vi "XY Graph Get Plot Properties.vi"(8 "Error In":errorcluster, 10 "Plot Idx":i32, 11 "XYGraph in":T1) -> (0 "Error Out":errorcluster, 2 "XY Plot Properties":T2, 3 "XYGraph out":T1, 4 "Plot.XScaleIdx":u32, 6 "Plot.YScaleIdx":u32)   [LabVIEW 2021, in "XY Graph Add-Ons.lvlib"]
uses:
  XY Graph Add-Ons.lvlib
  XY Graph Plot Properties.ctl
  XY Graph Refnum.ctl
panel:
  # "see the License on the block diagram (Ctrl+E or Window:Show Block Diagram)"
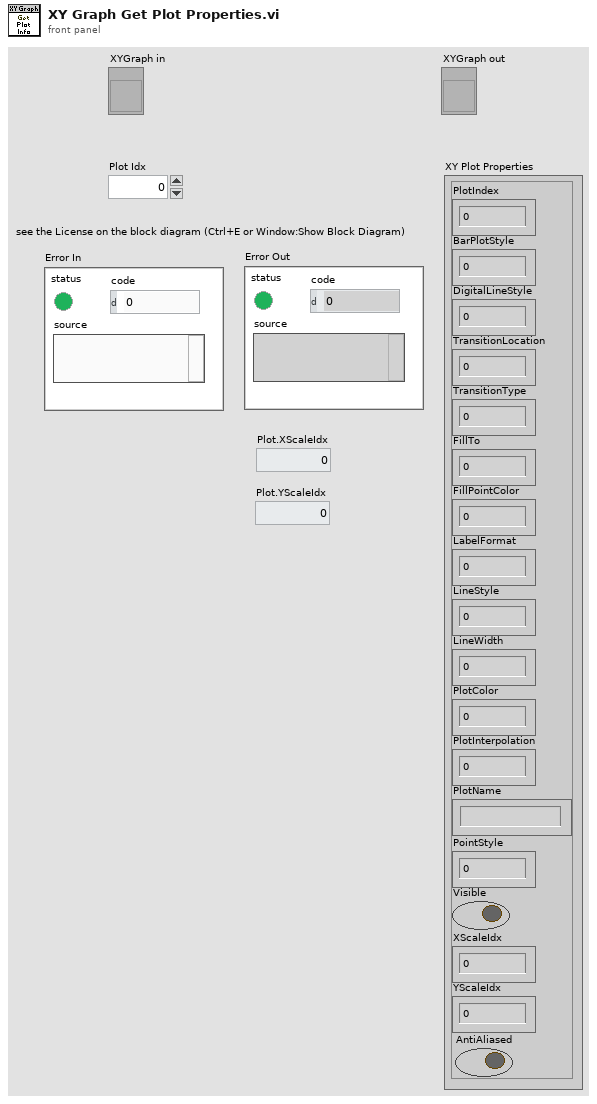
[diagram p1: front panel]
types:
  T1 = typedef "XY Graph Add-Ons.lvlib/XY Graph Refnum.ctl" = refnum<vi>
  T2 = typedef "XY Graph Add-Ons.lvlib/XY Graph Plot Properties.ctl" = cluster{"PlotIndex":i32, "BarPlotStyle":u8, "DigitalLineStyle":u8, "TransitionLocation":u8, "TransitionType":u8, "FillTo":i16, "FillPointColor":u32, "LabelFormat":u8, "LineStyle":u8, "LineWidth":u8, "PlotColor":u32, "PlotInterpolation":u8, "PlotName":string, "PointStyle":u8, "Visible":bool, "XScaleIdx":u32, "YScaleIdx":u32, "AntiAliased":bool}
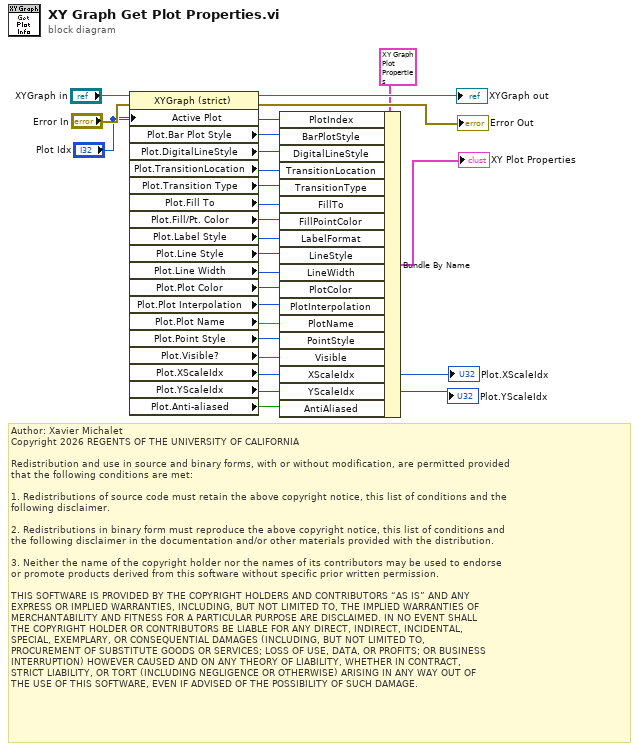
[diagram p0: block diagram]
diagram:
  # "Author: Xavier Michalet\nCopyright 2026 REGENTS OF THE UNIVERSITY OF CALIFORNIA\n\nRedistribution and use in source and binary forms, with or without modification, are permitted provided\nthat the following conditions are met:\n\n1. Redistributions of source code must retain the above copyright notice, this list of conditions and the\nfollowing disclaimer.\n\n2. Redistributions in binary form must reproduce the above copyright notice, this list of conditions and\nthe following disclaimer in the documentation and/or other materials provided with the distribution.\n\n3. Neither the name of the copyright holder nor the names of its contributors may be used to endorse \nor promote products derived from this software without specific prior written permission.\n\nTHIS SOFTWARE IS PROVIDED BY THE COPYRIGHT HOLDERS AND CONTRIBUTORS “AS IS” AND ANY \nEXPRESS OR IMPLIED WARRANTIES, INCLUDING, BUT NOT LIMITED TO, THE IMPLIED WARRANTIES OF\nMERCHANTABILITY AND FITNESS FOR A PARTICULAR PURPOSE ARE DISCLAIMED. IN NO EVENT SHALL\nTHE COPYRIGHT HOLDER OR CONTRIBUTORS BE LIABLE FOR ANY DIRECT, INDIRECT, INCIDENTAL, \nSPECIAL, EXEMPLARY, OR CONSEQUENTIAL DAMAGES (INCLUDING, BUT NOT LIMITED TO, \nPROCUREMENT OF SUBSTITUTE GOODS OR SERVICES; LOSS OF USE, DATA, OR PROFITS; OR BUSINESS\nINTERRUPTION) HOWEVER CAUSED AND ON ANY THEORY OF LIABILITY, WHETHER IN CONTRACT, \nSTRICT LIABILITY, OR TORT (INCLUDING NEGLIGENCE OR OTHERWISE) ARISING IN ANY WAY OUT OF\nTHE USE OF THIS SOFTWARE, EVEN IF ADVISED OF THE POSSIBILITY OF SUCH DAMAGE."
  n1 = property class="XYGraph (strict)"(reference="XYGraph in", error in="Error In", "Active Plot"="Plot Idx") -> (reference out=→"XYGraph out":T1, error out=→"Error Out":errorcluster, "Plot.Bar Plot Style"=w17:u8, "Plot.DigitalLineStyle"=w16:u8, "Plot.TransitionLocation"=w15:u8, "Plot.Transition Type"=w14:u8, "Plot.Fill To"=w13:i16, "Plot.Fill/Pt. Color"=w12:u32, "Plot.Label Style"=w11:u8, "Plot.Line Style"=w10:u8, "Plot.Line Width"=w9:u8, "Plot.Plot Color"=w8:u32, "Plot.Plot Interpolation"=w7:u8, "Plot.Plot Name"=w6:string, "Plot.Point Style"=w5:u8, "Plot.Visible?"=w4:bool, "Plot.XScaleIdx"=w2:u32, "Plot.YScaleIdx"=w1:u32, "Plot.Anti-aliased"=w3:bool)
  "Plot.XScaleIdx" <- w2
  "Plot.YScaleIdx" <- w1
  n2 = Bundle By Name(cluster=T2 {"PlotIndex"=0, "BarPlotStyle"=0, "DigitalLineStyle"=0, "TransitionLocation"=0, "TransitionType"=0, "FillTo"=0, "FillPointColor"=0, "LabelFormat"=0, "LineStyle"=0, "LineWidth"=0, "PlotColor"=0, "PlotInterpolation"=0, "PlotName"="", "PointStyle"=0, "Visible"=FALSE, "XScaleIdx"=0, "YScaleIdx"=0, "AntiAliased"=FALSE} ("XY Plot Properties"), "PlotIndex"="Plot Idx", "BarPlotStyle"=w17, "DigitalLineStyle"=w16, "TransitionLocation"=w15, "TransitionType"=w14, "FillTo"=w13, "FillPointColor"=w12, "LabelFormat"=w11, "LineStyle"=w10, "LineWidth"=w9, "PlotColor"=w8, "PlotInterpolation"=w7, "PlotName"=w6, "PointStyle"=w5, "Visible"=w4, "XScaleIdx"=w2, "YScaleIdx"=w1, "AntiAliased"=w3) -> (→"XY Plot Properties":T2)
